vi "StepBack.vi"(8 "Error":errorcluster, 11 "Tree in":refnum<class "Tree.lvclass">) -> (0 "Error":errorcluster, 1 "StepForward":T1(ring), 2 "StepBack":T1(ring), 3 "Tree out":refnum<class "Tree.lvclass">)   [LabVIEW 2021, in "Tree.lvlib" / "Tree.lvclass"]
uses:
  Tree.lvclass
  Private/TreeControllerTag.ctl
  Tree.lvclass/Tree.ctl
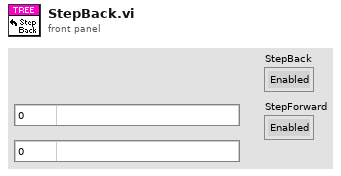
[diagram p1: front panel]
types:
  T1 = enum8{"Enabled", "Disabled", "Disabled and Grayed Out"}
  T2 = typedef "Tree.lvlib/Tree.lvclass/TreeControllerTag.ctl" = enum8{"Null", "1. Add item", "2. Delete item", "3. Get All Tree Data", "4. Drag Starting", "5. Drag Ended", "6. Add Tree Values", "7. Get Item Value", "8. Edit Item", "9. StepBack", "10. Filter"}
  T3 = cluster{"StepBack":enum8{"Enabled", "Disabled", "Disabled and Grayed Out"}, "StepForward":enum8{"Enabled", "Disabled", "Disabled and Grayed Out"}}
  T4 = cluster{"T=Back F=Forward":bool, "queue out":refnum<queue>}
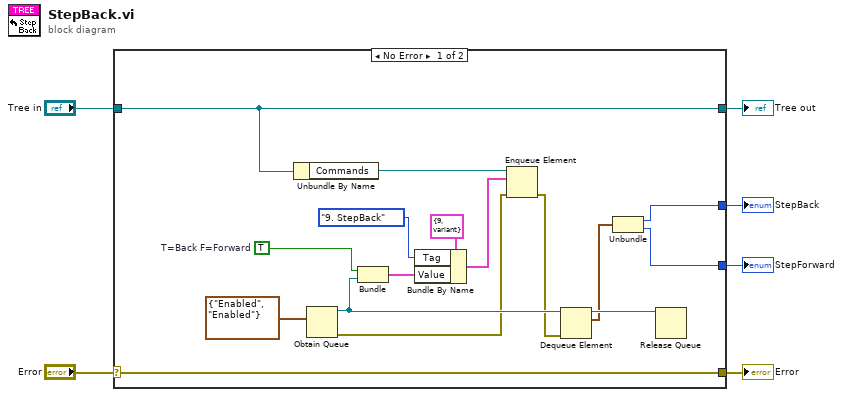
[diagram p0: block diagram]
diagram:
  n1 = case shown="No Error" "Error" {
    selector: "Error" -> [w22 w24]
    tunnel: [w22 w24] -> w5
    tunnel: [w19 w23] -> w3
    tunnel: "Tree in" -> [w19 w23]
    tunnel: [w11 _] -> w2
    tunnel: [w10 _] -> w1
    frame No Error {
      w16 = TRUE  # T=Back F=Forward
      n2 = Unbundle By Name(w19) -> ("Commands"=w21:refnum<queue>)
      n3 = Obtain Queue(element data type=T3 {"StepBack"=enum."Enabled", "StepForward"=enum."Enabled"}) -> (queue out=w14:refnum<queue>, error out=w8:errorcluster)  [unwired: 4 in, 1 out]
      n4 = Bundle("T=Back F=Forward"=w16, "queue out"=w14) -> (w15:T4)  [unwired: 1 in]
      n5 = Bundle By Name(cluster=cluster{"Tag":u8, "Value":variant} {"Tag"=9, "Value"=variant} ("element"), "Tag"=TreeControllerTag."9. StepBack", "Value"=w15) -> (w18:cluster{"Tag":u8, "Value":variant})
      n6 = Enqueue Element(queue=w21, element=w18, error in (no error)=w8) -> (error out=w9:errorcluster)  [unwired: 1 in, 2 out]
      n7 = Dequeue Element(queue=w14, error in (no error)=w9) -> (queue out=w13:refnum<queue>, element=w12:T3)  [unwired: 1 in, 2 out]
      n8 = Unbundle(w12) -> ("StepBack"=w10:T1, "StepForward"=w11:T1)
      n9 = Release Queue(queue=w13) -> ()  [unwired: 2 in, 3 out]
    }
    frame Error {
    }
  }
  "Error" <- w5
  "Tree out" <- w3
  "StepForward" <- w2
  "StepBack" <- w1
